vi "Check for Fresh Message.vi"(8 "error in":errorcluster, 11 "Handle PAS Vrange Request in":refnum<class "Handle PAS Vrange Request.lvclass">) -> (0 "error out":errorcluster, 1 "Enqueuer":refnum<class "Message Enqueuer.lvclass">, 2 "Enqueuer not Valid":bool, 3 "Handle PAS Vrange Request out":refnum<class "Handle PAS Vrange Request.lvclass">)   [LabVIEW 2014, in "Handle PAS Vrange Request.lvclass"]
doc: "This method is a dynamic method that \n1) checks for a good connection to the shared variable. If it is not present, then it attempts to connect If a connection is not available, then this VI will do nothing.\n2) Check the state of the enqueuer. If the state is no good, return with this indication and do nothing.\n2) If the connection is good, check to see if the current shared variable state has changed.\n3) If the state has changed, pump the message into the appropriate enqueuer."
uses:
  Handle PAS Vrange Request.lvclass
  <vilib>/ActorFramework/Message Enqueuer/Message Enqueuer.lvclass
  Instr Actor/Messages/Set Vrange MSG/Set Vrange MSG.lvclass
  Instr Actor/Messages/Set Vrange MSG/Set Vrange MSG.lvclass/Set Vrange MSG.ctl
  <vilib>/ActorFramework/Message Enqueuer/Message Enqueuer.lvclass/Message Enqueuer.ctl
  Instr Actor/Messages/Set Vrange MSG/Write Vrange.vi
  <vilib>/ActorFramework/Message Priority Queue/Priority Enqueue.vi
  Network Command Processor.lvclass
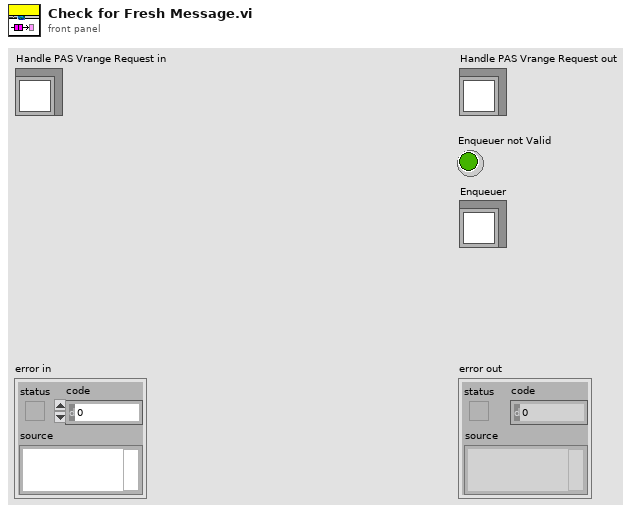
[diagram p1: front panel]
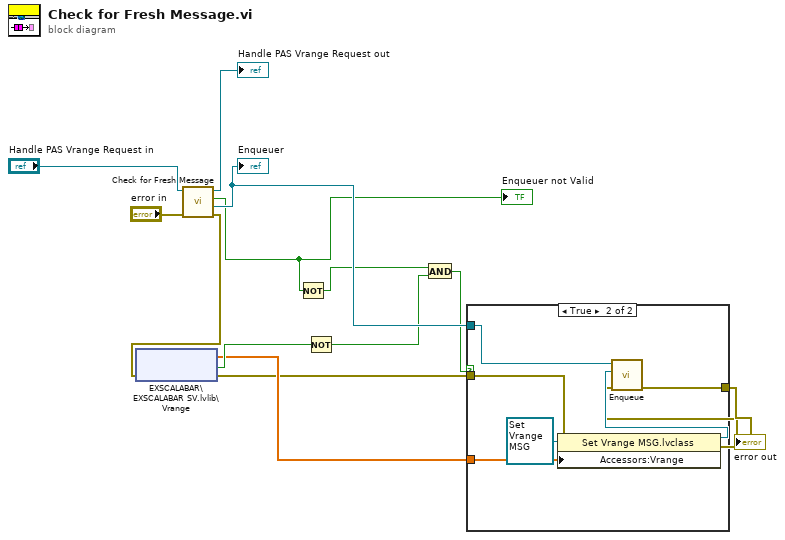
[diagram p0: block diagram]
diagram:
  n1 = call-parent "Check for Fresh Message.vi"("error in"="error in", "Network Command Processor in"="Handle PAS Vrange Request in") -> ("error out"=w3:errorcluster, "Enqueuer"=w10:refnum<class "Message Enqueuer.lvclass">, "Enqueuer not Valid"=w8:bool, "Network Command Processor out"=→"Handle PAS Vrange Request out":refnum<class "Handle PAS Vrange Request.lvclass">)  [unwired: 6 in]
  "Enqueuer not Valid" <- w8
  "Enqueuer" <- w10
  n2 = shared-variable "EXSCALABAR\\EXSCALABAR SV.lvlib\\Vrange"(error in=w3) -> (w4:sgl[], error out=w2:errorcluster, w9:bool)  [unwired: 1 in]
  n3 = Not(x=w8) -> (.not. x?=w7:bool)
  n4 = Not(x=w9) -> (.not. x?=w6:bool)
  n5 = And(x=w7, y=w6) -> (x .and. y?=w5:bool)
  n6 = case shown="True" w5 {
    tunnel: w10 -> [_ w18]
    tunnel: w4 -> [_ w20]
    tunnel: w2 -> [w14 w17]
    tunnel: [w14 w15] -> w1
    frame False {
    }
    frame True {
      n7 = property class="Set Vrange MSG.lvclass"(reference=refnum<class "Set Vrange MSG.lvclass"> refnum ("Instrument Lib:Set Vrange MSG.lvclass"), error in=w17, "Accessors:Vrange"=w20) -> (reference out=w19:refnum<class "Set Vrange MSG.lvclass">, error out=w16:errorcluster)
      n8 = call <vilib>:"Enqueue.vi"("error in (no error)"=w16, "Message"=w19, "Message Enqueuer in"=w18) -> ("error out"=w15:errorcluster)  [unwired: 7 in, 1 out]
    }
  }
  "error out" <- w1
